vi "Load INI Config_EStop.vi"(8 "error in":errorcluster, 11 "configuration file path":path) -> (0 "error out":errorcluster)   [LabVIEW 2021]
uses:
  DAQ_Data.ctl
  MUX_Data.ctl
  Keysight6700C_Data.ctl
  DMM_Data.ctl
  <vilib>/Utility/config.llb/Read Key (String).vi
  <vilib>/Utility/config.llb/NI_LVConfig.lvlib
panel:
  out "data":T1[](array[typedef])
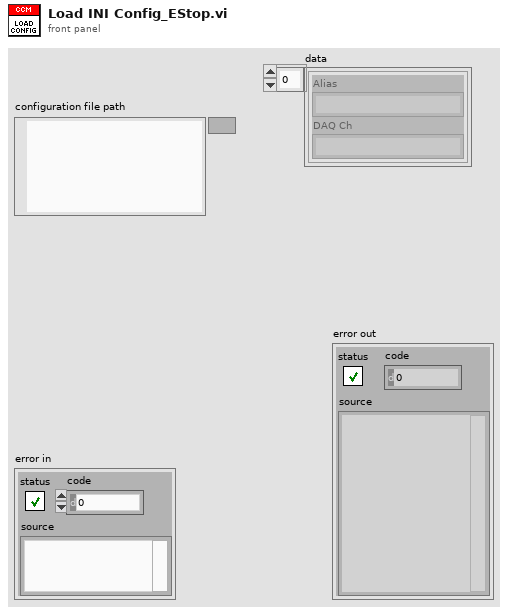
[diagram p1: front panel]
types:
  T1 = typedef "DAQ_Data.ctl" = cluster{"Alias":string, "DAQ Ch":string}
  T2 = typedef "NI_LVConfig.lvlib/Config Data RefNum.ctl" = refnum<k1>
  T3 = typedef "MUX_Data.ctl" = cluster{"Channel":string, "Topology":string}
  T4 = typedef "Keysight6700C_Data.ctl" = cluster{"Alias":string, "Device":string, "Channel name":string}
  T5 = typedef "DMM_Data.ctl" = cluster{"Channel":string, "MUX":string, "Route":string}
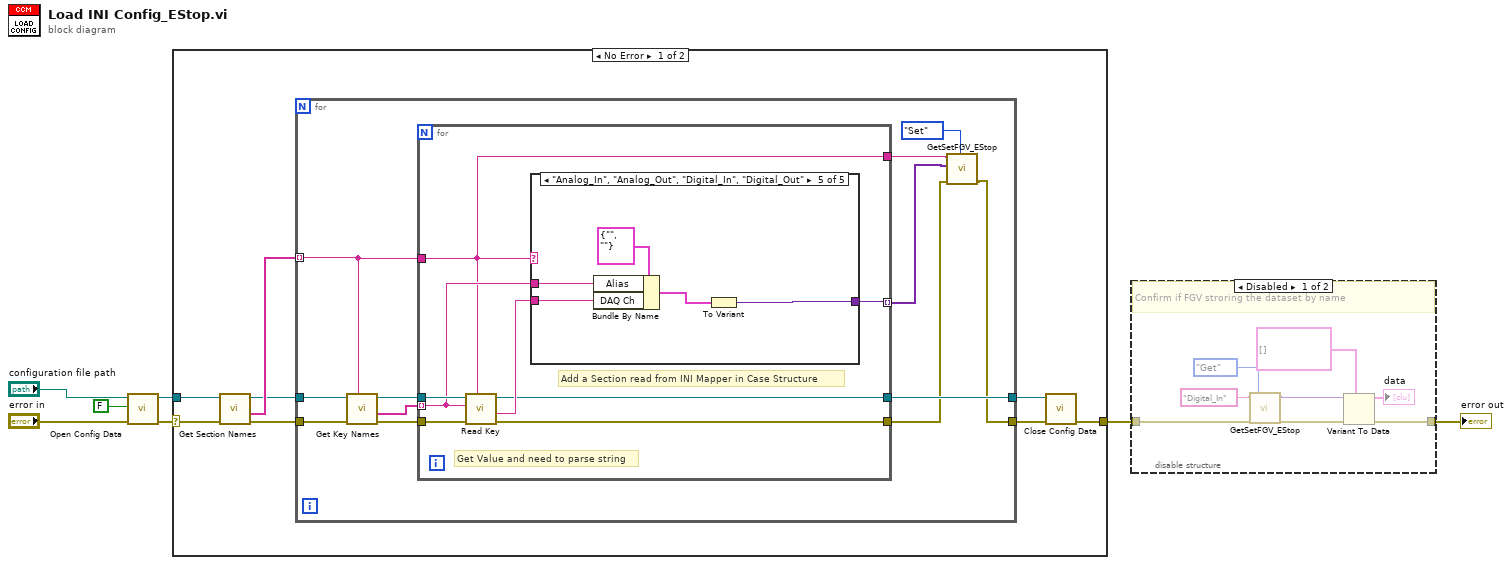
[diagram p0: block diagram]
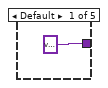
[diagram p2: hidden frame]
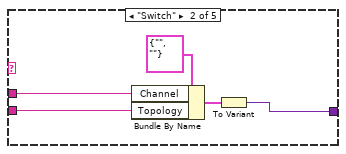
[diagram p3: hidden frame]
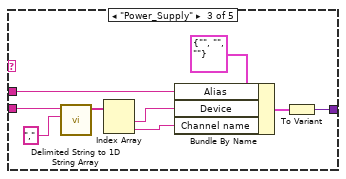
[diagram p4: hidden frame]
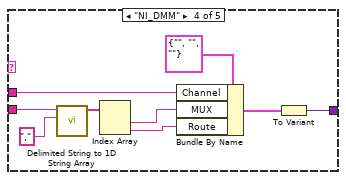
[diagram p5: hidden frame]
diagram:
  n1 = call <vilib>:"Open Config Data.vi"("error in (no error)"="error in", "create file if necessary (T)"=FALSE, "configuration file path"="configuration file path") -> ("error out"=w5:errorcluster, "refnum"=w6:T2)  [unwired: 6 in, 1 out]
  n2 = case shown="No Error" w5 {
    selector: w5 -> [w15 w65]
    tunnel: [w8 w65] -> w3
    tunnel: w6 -> [w14 _]
    frame No Error {
      n3 = call <vilib>:"Get Section Names.vi"("error in (no error)"=w15, "refnum"=w14) -> ("error out"=w12:errorcluster, "section names"=w13:string[], "refnum out"=w11:T2)  [unwired: 7 in]
      n4 = for {
        tunnel: w13 -> [w24] mode=indexing
        tunnel: w12 -> [w27]
        tunnel: w11 -> [w26]
        tunnel: [w25] -> w10
        tunnel: [w19] -> w9
        n5 = call <vilib>:"Get Key Names.vi"("section"=w24, "error in (no error)"=w27, "refnum"=w26) -> ("error out"=w23:errorcluster, "key names"=w22:string[], "refnum out"=w21:T2)  [unwired: 5 in, 1 out]
        n6 = for {
          tunnel: w22 -> [w32] mode=indexing
          tunnel: w24 -> [w28]
          tunnel: w21 -> [w34]
          tunnel: [w30] -> w25
          tunnel: [w29] -> w18 mode=indexing
          tunnel: w23 -> [w35]
          tunnel: [w33] -> w20
          tunnel: [w28] -> w17
          # "Add a Section read from INI Mapper in Case Structure"
          # "Get Value and need to parse string"
          n7 = call-poly <vilib>:"Read Key.vi"("section"=w28, "error in (no error)"=w35, "key"=w32, "refnum"=w34) -> ("error out"=w33:errorcluster, "value"=w31:string, "refnum out"=w30:T2)  [unwired: 4 in, 1 out]
          n8 = case shown="\"Analog_In\", \"Analog_Out\", \"Digital_In\", \"Digital_Out\"" w28 {
            tunnel: w32 -> [_ w40 w48 w53 w62]
            tunnel: w31 -> [_ w39 w44 w56 w61]
            tunnel: [variant ("Variant") w38 w50 w54 w64] -> w29
            frame Default {
            }
            frame "Switch" {
              n9 = Bundle By Name(cluster=T3 {"Channel"="", "Topology"=""}, "Channel"=w40, "Topology"=w39) -> (w37:T3)
              n10 = To Variant(anything=w37) -> (Variant=w38:variant)
            }
            frame "Power_Supply" {
              n11 = call <vilib>:"Delimited String to 1D String Array.vi"("delimiter"=",", "delimited string"=w44) -> ("string array"=w46:string[])  [unwired: 9 in]
              n12 = Index Array(array=w46) -> (element #1=w43:string, element #2=w42:string)  [unwired: 2 in]
              n13 = Bundle By Name(cluster=T4 {"Alias"="", "Device"="", "Channel name"=""} ("DAQ Data"), "Alias"=w48, "Device"=w43, "Channel name"=w42) -> (w47:T4)
              n14 = To Variant(anything=w47) -> (Variant=w50:variant)
            }
            frame "NI_DMM" {
              n15 = call <vilib>:"Delimited String to 1D String Array.vi"("delimiter"=",", "delimited string"=w56) -> ("string array"=w58:string[])  [unwired: 9 in]
              n16 = Index Array(array=w58) -> (element #1=w52:string, element #2=w51:string)  [unwired: 2 in]
              n17 = Bundle By Name(cluster=T5 {"Channel"="", "MUX"="", "Route"=""} ("DAQ Data"), "Channel"=w53, "MUX"=w52, "Route"=w51) -> (w55:T5)
              n18 = To Variant(anything=w55) -> (Variant=w54:variant)
            }
            frame "Analog_In", "Analog_Out", "Digital_In", "Digital_Out" {
              n19 = Bundle By Name(cluster=T1 {"Alias"="", "DAQ Ch"=""} ("DAQ Data"), "Alias"=w62, "DAQ Ch"=w61) -> (w60:T1)
              n20 = To Variant(anything=w60) -> (Variant=w64:variant)
            }
          }
        }
        n21 = call "GetSetFGV_EStop.vi"("Method (Get)"=enum16{"Get", "Set"}."Set", "error in"=w20, "Data In"=w18, "Name"=w17) -> ("error out"=w19:errorcluster)  [unwired: 6 in, 1 out]
      }
      n22 = call <vilib>:"Close Config Data.vi"("error in (no error)"=w9, "refnum"=w10) -> ("error out"=w8:errorcluster)  [unwired: 8 in, 1 out]
    }
    frame Error {
    }
  }
  n23 = disable-structure "Diagram Disable Structure" shown="Disabled" {
    disable-tunnel: w3 -> [w70 w74]
    disable-tunnel: [w73 w74] -> w2
    frame Disabled {
      # "Confirm if FGV stroring the dataset by name"
      n24 = call "GetSetFGV_EStop.vi"("Method (Get)"=enum16{"Get", "Set"}."Get", "error in"=w70, "Name"="Digital_In") -> ("error out"=w69:errorcluster, "Data out"=w68:variant)  [unwired: 7 in]
      n25 = Variant To Data(error in=w69, type=T1[] [], Variant=w68) -> (data=→"data":T1[], error out=w73:errorcluster)
    }
    frame Enabled {
      # "Enble this for production"
    }
  }
  "error out" <- w2
